vi "Read Incoming Bytes.vi"(8 "error in (no error)":errorcluster, 9 "timeout (1000 ms)":i32=1000, 10 "bytes to read (100)":i32=100, 11 "Connection in":refnum<class "Connection.lvclass">) -> (0 "error out":errorcluster, 1 "timed out":bool, 2 "Bytes":u8[](array[numeric]) format="%08b", 3 "Connection out":refnum<class "Connection.lvclass">, 4 "connected":bool)   [LabVIEW 2013, in "MQTT_Connection.lvlib" / "Connection.lvclass"]
uses:
  Connection.lvclass
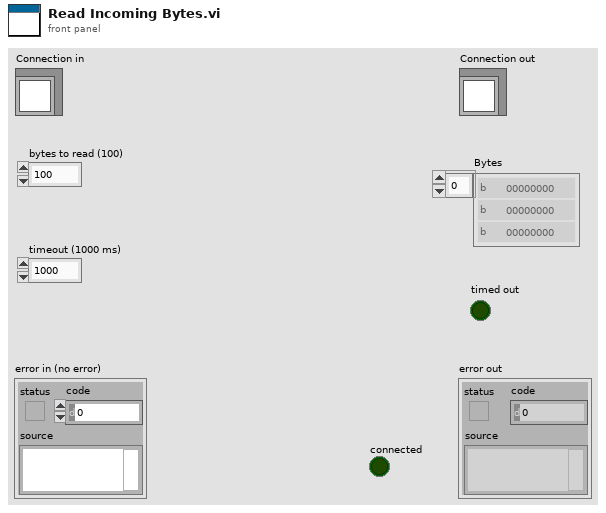
[diagram p1: front panel]
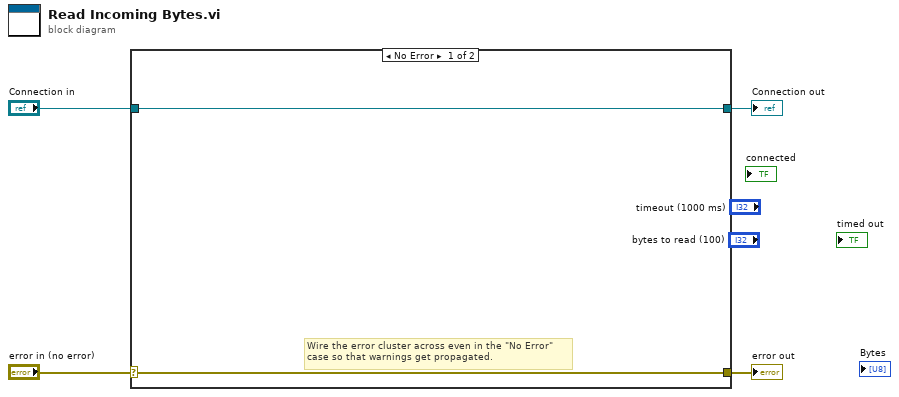
[diagram p0: block diagram]
diagram:
  n1 = case shown="No Error" "error in (no error)" {
    selector: "error in (no error)" -> [w5 w8]
    tunnel: [w5 w8] -> w3
    tunnel: [w6 w7] -> w1
    tunnel: "Connection in" -> [w6 w7]
    frame No Error {
      # "Wire the error cluster across even in the \"No Error\"\ncase so that warnings get propagated."
    }
    frame Error {
    }
  }
  "error out" <- w3
  "Connection out" <- w1
